vi "Main.vi"(8 "error in":errorcluster, 11 "DS TCP Server in":refnum<class "DS TCP Server.lvclass">) -> (0 "error out":errorcluster, 3 "DS TCP Server out":refnum<class "DS TCP Server.lvclass">)   [LabVIEW 2017, in "DS TCP Server.lvlib" / "DS TCP Server.lvclass"]
doc: "The <b>Queued Message Handler</b> of the Worker that owns this VI."
uses:
  DS TCP Server.lvclass
  C:/Program Files (x86)/National Instruments/LabVIEW 2017/vi.lib/addons/_Workers/Library/Classes/Worker/Worker.lvclass
  DS TCP Server.lvclass/DS TCP Server.ctl
  Initialization Data.ctl
  Response Cases.ctl
  <vilib>/addons/_Workers/Library/Case Label.ctl
  rqp_Send Data to Debug Client.ctl
  Common VIs/DC_UID.ctl
  <vilib>/addons/_Workers/Library/Classes/Message/Priority.ctl
  rqp_Start Listening.ctl
  <vilib>/addons/_Workers/Library/Classes/Message Queue/Message Queue.lvclass
  DS TCP Listener/rqp_Listen for Connections.ctl
  rqp_Message Log Ready.ctl
  Common VIs/Message Log ID.ctl
  Message Log Data.ctl
  rqp_Message Log Exited.ctl
  rsp_Server Port Open.ctl
  rsp_Connection Notify.ctl
  <vilib>/Utility/error.llb/Error Cluster From Error Code.vi
  <vilib>/ErrorRing/Error Ring.xnode
  DS TCP Listener/DS TCP Listener.lvclass
  <vilib>/addons/_Workers/Library/Workers.lvlib
  DS TCP Read/DS TCP Read.lvclass
  <vilib>/addons/_Workers/Library/Classes/Message/Message.lvclass
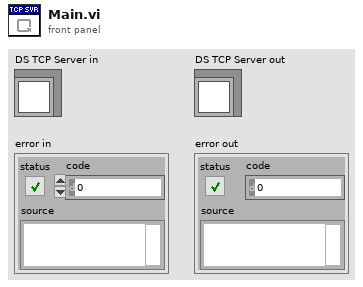
[diagram p1: front panel]
types:
  T1 = typedef "DS TCP Server.lvlib/DS TCP Server.lvclass/Initialization Data.ctl" = cluster{"Response Cases":T2}
  T2 = typedef "DS TCP Server.lvlib/DS TCP Server.lvclass/Response Cases.ctl" = cluster{"Server Port Open":T3, "Connection Notify":T3, "Incompatible DC Connection":T3}
  T3 = typedef "Workers.lvlib/Case Label.ctl" = string
  T4 = typedef "DS TCP Server.lvlib/DS TCP Server.lvclass/rqp_Send Data to Debug Client.ctl" = cluster{"DC_UID":T5, "String to send":string}
  T5 = typedef "DC_UID.ctl" = string
  T6 = typedef "Workers.lvlib/Message.lvclass/Priority.ctl" = enum16{"Low", "Normal", "High"}
  T7 = typedef "DS TCP Server.lvlib/DS TCP Listener.lvclass/rqp_Listen for Connections.ctl" = cluster{"Server Name":string, "Port":u16}
  T8 = typedef "DS TCP Server.lvlib/DS TCP Server.lvclass/rqp_Start Listening.ctl" = cluster{"Server Name":string, "Port":u16, "App Manager Q":refnum<class "Message Queue.lvclass">}
  T9 = typedef "DS TCP Server.lvlib/DS TCP Server.lvclass/rqp_Message Log Ready.ctl" = cluster{"Message Log Q":refnum<class "Message Queue.lvclass">, "Message Log ID":T10, "DC_UID":T5}
  T10 = typedef "Message Log ID.ctl" = cluster{"Head Worker ID":string, "IP Address":string}
  T11 = typedef "DS TCP Server.lvlib/DS TCP Server.lvclass/Message Log Data.ctl" = cluster{"Message Log Q":refnum<class "Message Queue.lvclass">, "Message Log ID":T10, "DC_UID":T5}
  T12 = typedef "DS TCP Server.lvlib/DS TCP Server.lvclass/rqp_Message Log Exited.ctl" = cluster{"DC_UID":T5}
  T13 = typedef "DS TCP Server.lvlib/DS TCP Server.lvclass/rsp_Server Port Open.ctl" = cluster{"Port":u16}
  T14 = typedef "DS TCP Server.lvlib/DS TCP Server.lvclass/rsp_Connection Notify.ctl" = cluster{"Connected?":bool, "DC_UID":T5, "Message Priority":T6, "IP Address":string}
  T15 = typedef "DS TCP Server.lvlib/DS TCP Server.lvclass/Connection ID.ctl" = cluster{"Connection Ref":refnum<k5>, "DC_UID":T5, "Message Priority":T6, "IP Address":string}
  T16 = typedef "DS TCP Server.lvlib/DS TCP Listener.lvclass/rsp_Add Listener.ctl" = cluster{"listener ID":refnum<k5>, "Port":u16}
  T17 = typedef "DS TCP Server.lvlib/DS TCP Read.lvclass/rsp_Connection Lost.ctl" = cluster{"connection ID out":refnum<k5>, "Message Queue":refnum<class "Message Queue.lvclass">}
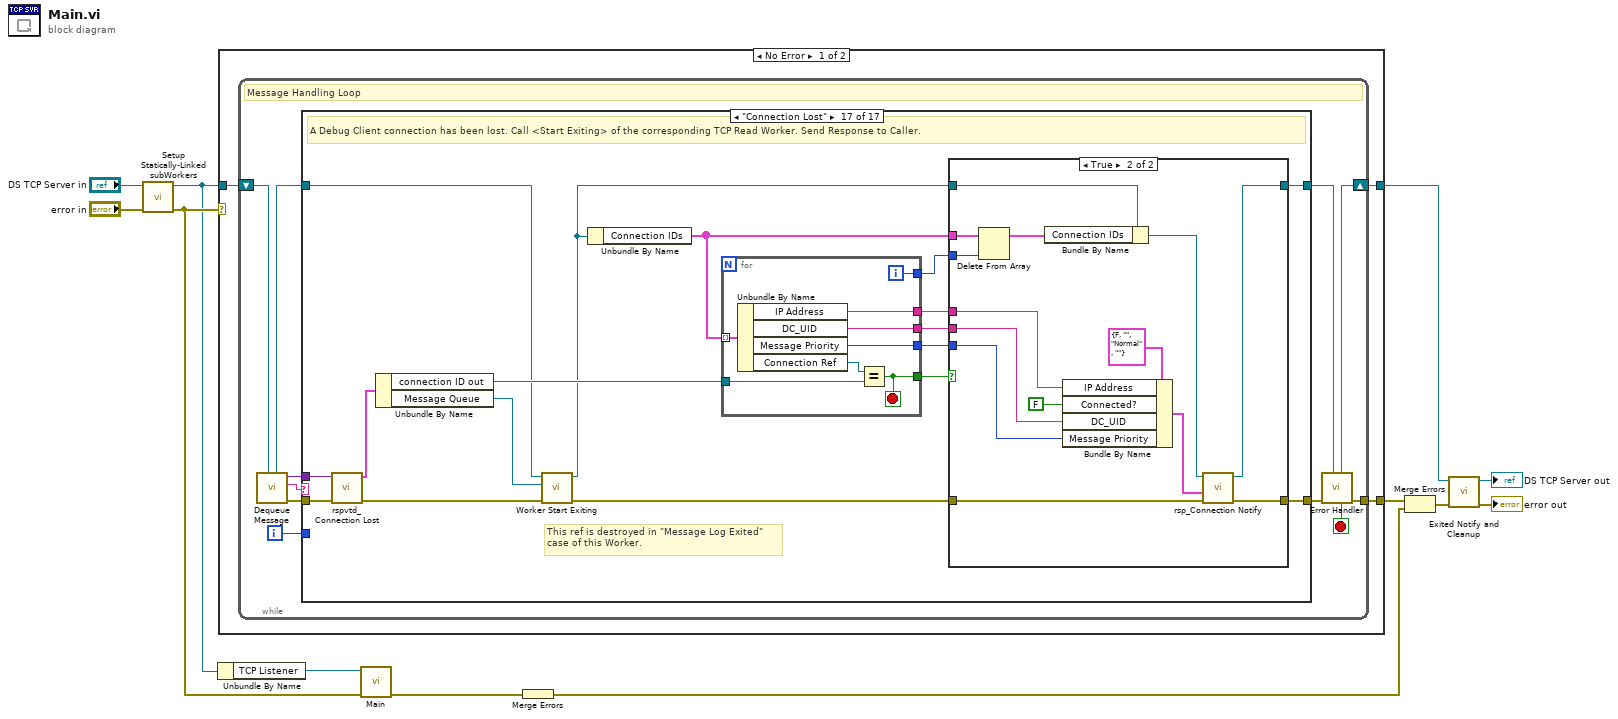
[diagram p0: block diagram]
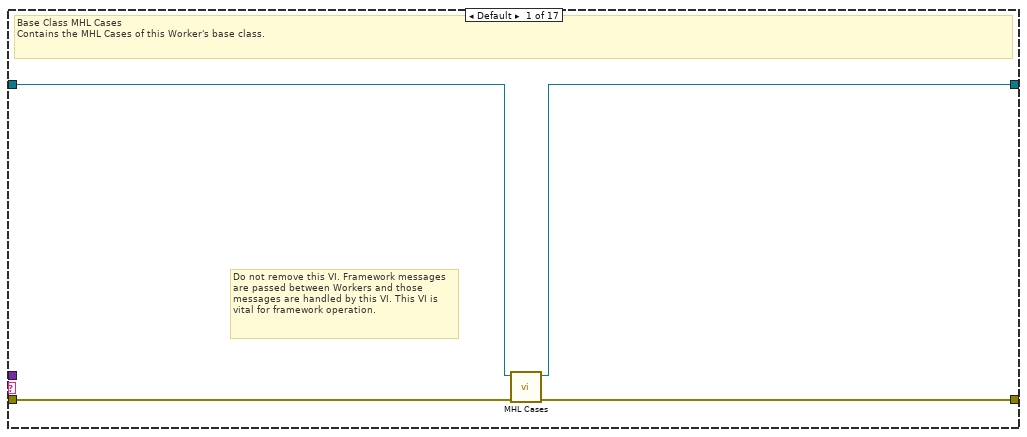
[diagram p2: hidden frame]
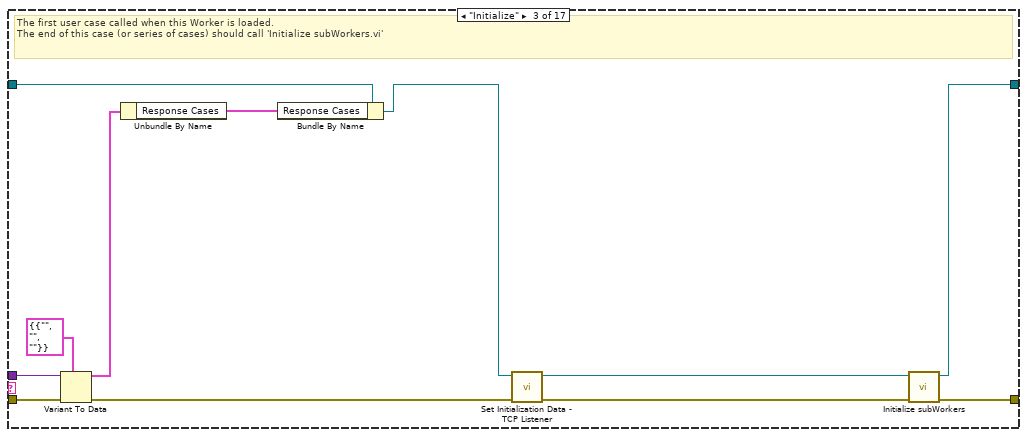
[diagram p4: hidden frame]
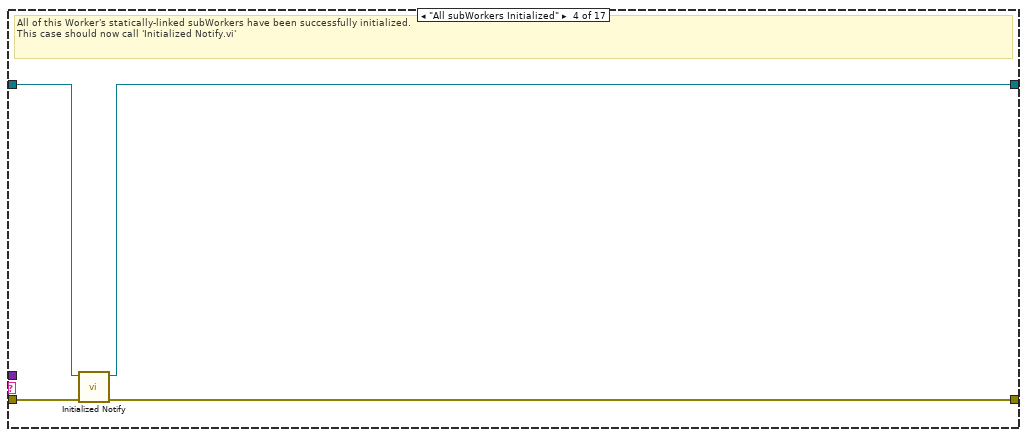
[diagram p5: hidden frame]
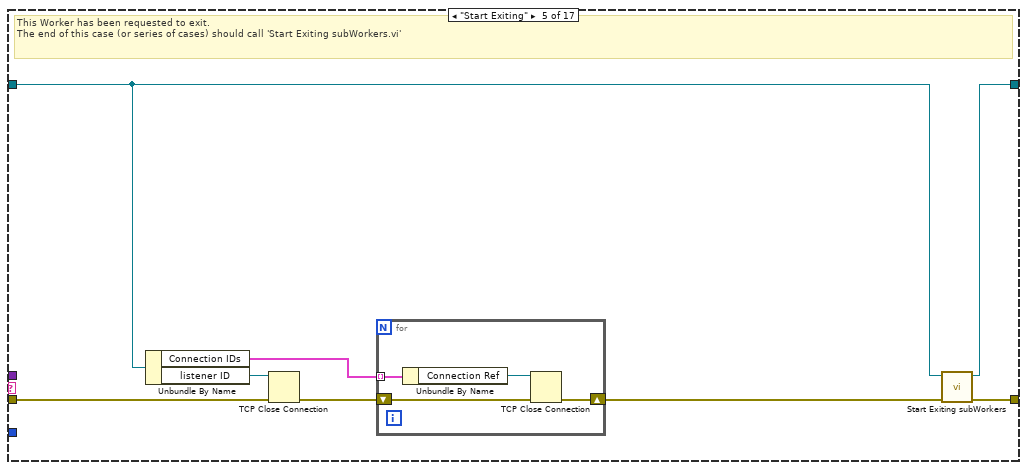
[diagram p6: hidden frame]
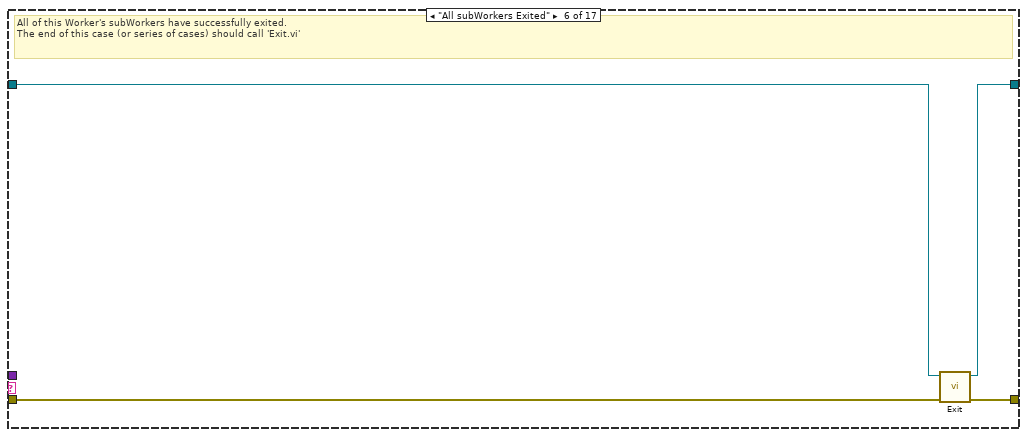
[diagram p7: hidden frame]
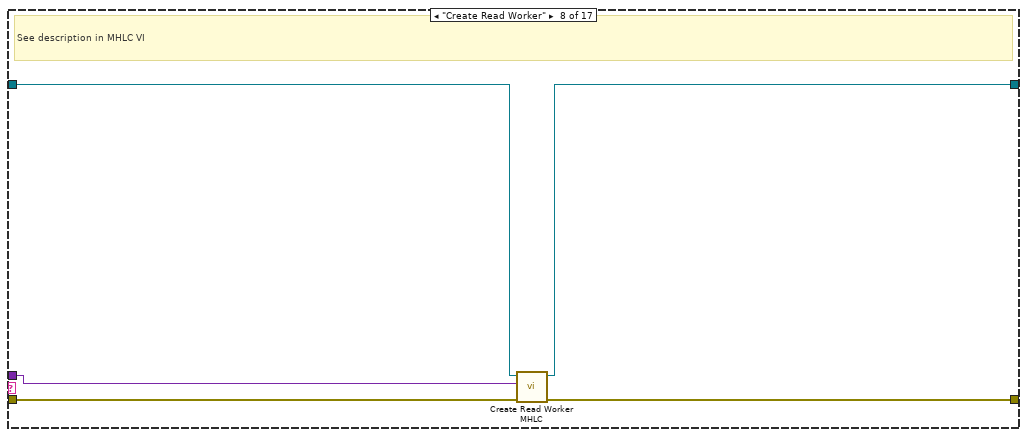
[diagram p9: hidden frame]
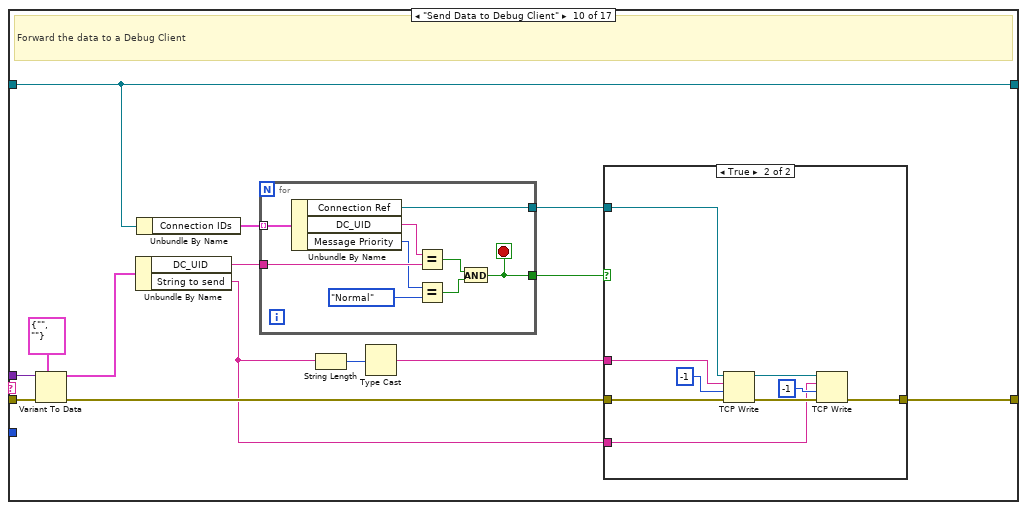
[diagram p11: hidden frame]
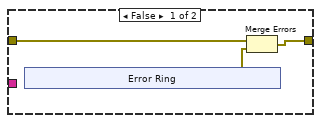
[diagram p12: hidden frame]
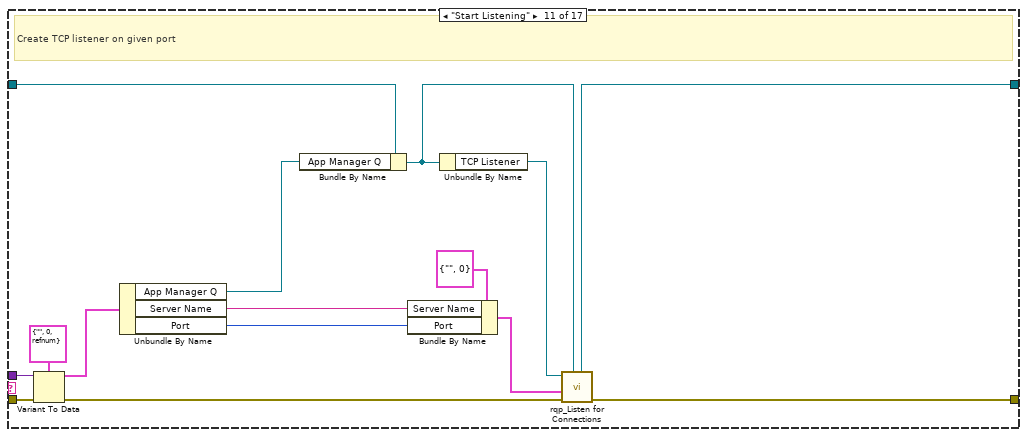
[diagram p13: hidden frame]
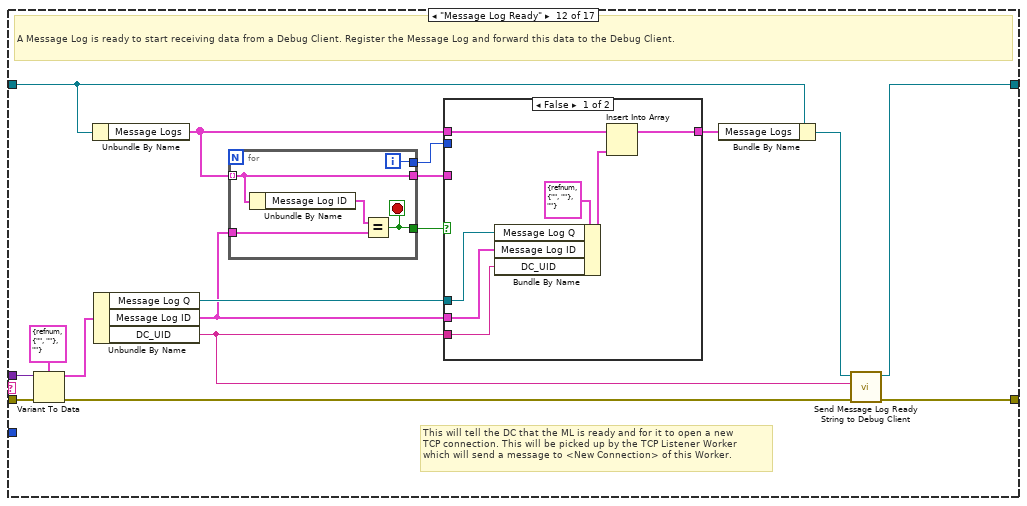
[diagram p14: hidden frame]
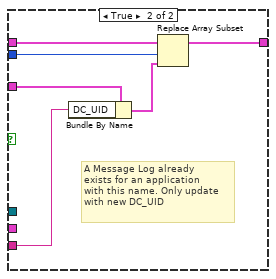
[diagram p15: hidden frame]
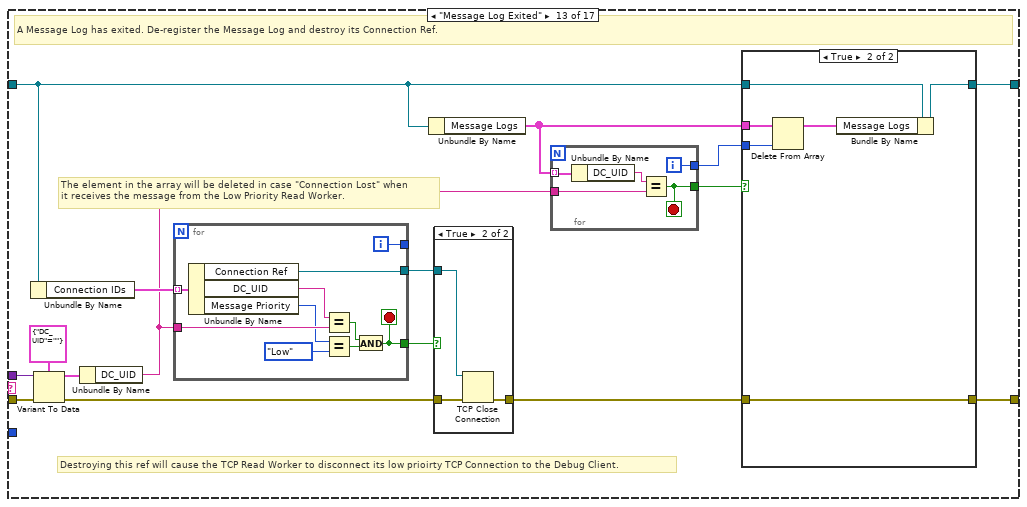
[diagram p16: hidden frame]
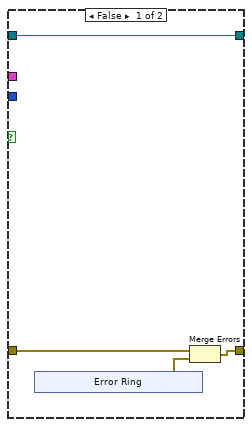
[diagram p17: hidden frame]
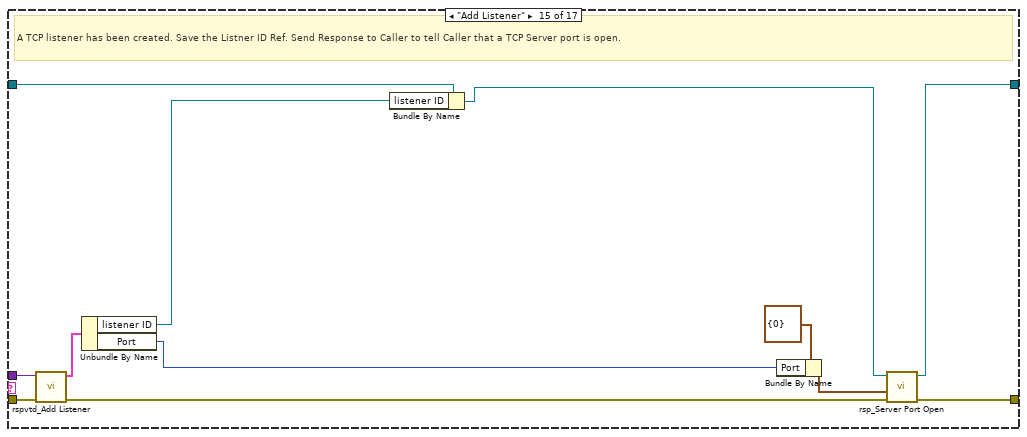
[diagram p20: hidden frame]
diagram:
  n1 = call "Setup Statically-Linked subWorkers.vi"("error in"="error in", "TCP Server in"="DS TCP Server in") -> ("error out"=w10:errorcluster, "TCP Server out"=w6:refnum<class "DS TCP Server.lvclass">)  [unwired: 8 in]
  n2 = Unbundle By Name(w6) -> ("TCP Listener"=w1:refnum<class "DS TCP Listener.lvclass">)
  n3 = case shown="No Error" w10 {
    tunnel: w6 -> [w15 w282]
    tunnel: [w13 w283] -> w9
    tunnel: [w14 w281] -> w11
    selector: w10 -> [_ w284]
    frame No Error {
      n4 = while {
        shift-right: [w24] -> w14
        shift-left: w15 -> [w26]
        tunnel: [w25] -> w13
        i -> [w17]
        stop <- w18 stop-if-true
        # "Message Handling Loop"
        n5 = call-dynamic "Dequeue Message.vi"("Worker"=w26) -> ("error out"=w23:errorcluster, "Case out"=w19:string, "Data out"=w16:variant, "Worker out"=w21:refnum<class "DS TCP Server.lvclass">)  [unwired: 6 in, 1 out]
        n6 = case "Worker MHL Case Structure (DO NOT CHANGE LABEL NAME)" shown="\"Connection Lost\"" w19 {
          tunnel: w23 -> [w30 w31 w42 w48 w54 w64 w66 w71 w73 w84 w128 w145 w179 w215 w225 w229 w239]
          tunnel: [w29 w31 w44 w46 w56 w63 w66 w69 w73 w77 w123 w140 w167 w215 w223 w230 w245] -> w22
          tunnel: w21 -> [w28 w32 w35 w47 w53 w61 w65 w67 w72 w82 w121 w138 w169 w214 w227 w232 w235]
          tunnel: [w27 w32 w43 w45 w55 w62 w65 w68 w72 w82 w122 w139 w170 w214 w224 w231 w244] -> w20
          tunnel: w17 -> [_ _ _ _ _ _ _ _ _ _ _ _ _ _ _ _ _]
          tunnel: w16 -> [_ _ w37 _ _ _ _ w70 _ w83 w125 w142 w177 _ w226 w228 w246]
          frame Default {
            # "Do not remove this VI. Framework messages are passed between Workers and those messages are handled by this VI. This VI is vital for framework operation."
            # "Base Class MHL Cases\nContains the MHL Cases of this Worker's base class."
            n7 = call-dynamic "MHL Cases.vi"("error in"=w30, "Worker in"=w28) -> ("error out"=w29:errorcluster, "Worker out"=w27:refnum<class "DS TCP Server.lvclass">)  [unwired: 8 in]
          }
          frame "------------ FRAMEWORK CASES -----------" {
            # "Start of Workers Framework Cases"
          }
          frame "Initialize" {
            # "The first user case called when this Worker is loaded.\nThe end of this case (or series of cases) should call 'Initialize subWorkers.vi'"
            n8 = Variant To Data(error in=w42, type=T1 {"Response Cases"={"Server Port Open"="", "Connection Notify"="", "Incompatible DC Connection"=""}} ("Initialization Data"), Variant=w37) -> (data=w34:T1, error out=w39:errorcluster)
            n9 = Unbundle By Name(w34) -> ("Response Cases"=w36:T2)
            n10 = Bundle By Name(cluster=w35, "Response Cases"=w36) -> (w33:refnum<class "DS TCP Server.lvclass">)
            n11 = call "Set Initialization Data - TCP Listener.vi"("error in"=w39, "TCP Server in"=w33) -> ("error out"=w41:errorcluster, "TCP Server out"=w40:refnum<class "DS TCP Server.lvclass">)  [unwired: 8 in]
            n12 = call-dynamic "Initialize subWorkers.vi"("error in"=w41, "Worker"=w40) -> ("error out"=w44:errorcluster, "dup Worker out"=w43:refnum<class "DS TCP Server.lvclass">)  [unwired: 8 in]
          }
          frame "All subWorkers Initialized" {
            # "All of this Worker's statically-linked subWorkers have been successfully initialized.\nThis case should now call 'Initialized Notify.vi'"
            n13 = call-dynamic "Initialized Notify.vi"("error in"=w48, "Worker"=w47) -> ("error out"=w46:errorcluster, "dup Worker out"=w45:refnum<class "DS TCP Server.lvclass">)  [unwired: 8 in]
          }
          frame "Start Exiting" {
            # "This Worker has been requested to exit. \nThe end of this case (or series of cases) should call 'Start Exiting subWorkers.vi'"
            n14 = Unbundle By Name(w53) -> ("Connection IDs"=w51:T15[], "listener ID"=w52:refnum<k5>)
            n15 = TCP Close Connection(connection ID=w52, error in (no error)=w54) -> (error out=w50:errorcluster)  [unwired: 1 in, 1 out]
            n16 = for {
              shift-right: [w59] -> w49
              shift-left: w50 -> [w60]
              tunnel: w51 -> [w58] mode=indexing
              n17 = Unbundle By Name(w58) -> ("Connection Ref"=w57:refnum<k5>)
              n18 = TCP Close Connection(connection ID=w57, error in (no error)=w60) -> (error out=w59:errorcluster)  [unwired: 1 in, 1 out]
            }
            n19 = call-dynamic "Start Exiting subWorkers.vi"("error_in"=w49, "Worker"=w53) -> ("error out"=w56:errorcluster, "dup Worker out"=w55:refnum<class "DS TCP Server.lvclass">)  [unwired: 8 in]
          }
          frame "All subWorkers Exited" {
            # "All of this Worker's subWorkers have successfully exited. \nThe end of this case (or series of cases) should call 'Exit.vi'"
            n20 = call-dynamic "Exit.vi"("error_in"=w64, "Worker"=w61) -> ("error out"=w63:errorcluster, "dup Worker out"=w62:refnum<class "DS TCP Server.lvclass">)  [unwired: 8 in]
          }
          frame "------------- LOCAL API CASES -------------" {
            # "Start of Workers Local API Cases"
          }
          frame "Create Read Worker" {
            # "See description in MHLC VI"
            n21 = call "Create Read Worker MHLC.vi"("error in (no error)"=w71, "Data in"=w70, "TCPServer in"=w67) -> ("error out"=w69:errorcluster, "TCPServer out"=w68:refnum<class "DS TCP Server.lvclass">)  [unwired: 7 in]
          }
          frame "------------- PUBLIC API CASES -------------" {
            # "Start of Public API Cases"
          }
          frame "Send Data to Debug Client" {
            # "Forward the data to a Debug Client"
            n22 = Variant To Data(error in=w84, type=T4 {"DC_UID"="", "String to send"=""} ("Data"), Variant=w83) -> (data=w81:T4, error out=w78:errorcluster)
            n23 = Unbundle By Name(w81) -> ("DC_UID"=w80:T5, "String to send"=w75:string)
            n24 = Unbundle By Name(w82) -> ("Connection IDs"=w87:T15[])
            n25 = for {
              tunnel: w87 -> [w113] mode=indexing
              tunnel: w80 -> [w111]
              tunnel: [w110] -> w74
              tunnel: [w105] -> w79
              stop <- w105 stop-if-true
              n26 = Unbundle By Name(w113) -> ("Connection Ref"=w110:refnum<k5>, "DC_UID"=w112:T5, "Message Priority"=w109:T6)
              n27 = Equal?(x=w112, y=w111) -> (x = y?=w107:bool)
              n28 = Equal?(x=w109, y=Priority."Normal") -> (x = y?=w106:bool)
              n29 = And(x=w107, y=w106) -> (x .and. y?=w105:bool)
            }
            n30 = String Length(string=w75) -> (length=w86:i32)
            n31 = Type Cast(x=w86) -> (*(type *) &x=w76:string)  [unwired: 1 in]
            n32 = case shown="True" w79 {
              tunnel: w78 -> [w90 w100]
              tunnel: [w89 w99] -> w77
              tunnel: w76 -> [_ w98]
              tunnel: w75 -> [_ w97]
              tunnel: w74 -> [_ w96]
              frame False {
                n33 = xnode "Error Ring"() -> ("error out"=w88:errorcluster)
                n34 = Merge Errors(w90, w88) -> (w89:errorcluster)
              }
              frame True {
                n35 = TCP Write(connection ID=w96, data in=w98, error in (no error)=w100, 9:-1 ("timeout ms (25000)")) -> (connection ID out=w102:refnum<k5>, error out=w101:errorcluster)  [unwired: 1 out]
                n36 = TCP Write(connection ID=w102, data in=w97, error in (no error)=w101, 9:-1 ("timeout ms (25000)")) -> (error out=w99:errorcluster)  [unwired: 2 out]
              }
            }
          }
          frame "Start Listening" {
            # "Create TCP listener on given port"
            n37 = Variant To Data(error in=w128, type=T8 {"Server Name"="", "Port"=0, "App Manager Q"=refnum} ("Data"), Variant=w125) -> (data=w124:T8, error out=w127:errorcluster)
            n38 = Unbundle By Name(w124) -> ("App Manager Q"=w114:refnum<class "Message Queue.lvclass">, "Server Name"=w117:string, "Port"=w116:u16)
            n39 = Bundle By Name(cluster=w121, "App Manager Q"=w114) -> (w115:refnum<class "DS TCP Server.lvclass">)
            n40 = Bundle By Name(cluster=T7 {"Server Name"="", "Port"=0} ("Data"), "Server Name"=w117, "Port"=w116) -> (w118:T7)
            n41 = Unbundle By Name(w115) -> ("TCP Listener"=w120:refnum<class "DS TCP Listener.lvclass">)
            n42 = call "rqp_Listen for Connections.vi"("Caller in"=w115, "error in"=w127, "Data"=w118, "DS TCP Listener in"=w120) -> ("error out"=w123:errorcluster, "dup Caller out"=w122:refnum<class "DS TCP Server.lvclass">)  [unwired: 5 in, 1 out]
          }
          frame "Message Log Ready" {
            # "This will tell the DC that the ML is ready and for it to open a new\nTCP connection. This will be picked up by the TCP Listener Worker\nwhich will send a message to <New Connection> of this Worker."
            # "A Message Log is ready to start receiving data from a Debug Client. Register the Message Log and forward this data to the Debug Client."
            n43 = Variant To Data(error in=w145, type=T9 {"Message Log Q"=refnum, "Message Log ID"={"Head Worker ID"="", "IP Address"=""}, "DC_UID"=""} ("Data"), Variant=w142) -> (data=w141:T9, error out=w144:errorcluster)
            n44 = Unbundle By Name(w138) -> ("Message Logs"=w134:T11[])
            n45 = Unbundle By Name(w141) -> ("Message Log Q"=w137:refnum<class "Message Queue.lvclass">, "Message Log ID"=w133:T10, "DC_UID"=w131:T5)
            n46 = for {
              tunnel: w134 -> [w159] mode=indexing
              tunnel: w133 -> [w162]
              tunnel: [w161] -> w132
              tunnel: [w160] -> w129
              tunnel: [w159] -> w130
              i -> [w160]
              stop <- w161 stop-if-true
              n47 = Unbundle By Name(w159) -> ("Message Log ID"=w163:T10)
              n48 = Equal?(x=w163, y=w162) -> (x = y?=w161:bool)
            }
            n49 = case shown="False" w132 {
              tunnel: w137 -> [w150 _]
              tunnel: [w149 w157] -> w135
              tunnel: w134 -> [w148 w158]
              tunnel: w133 -> [w147 _]
              tunnel: w131 -> [w146 w155]
              tunnel: w130 -> [_ w156]
              tunnel: w129 -> [_ w153]
              frame False {
                n50 = Bundle By Name(cluster=T11 {"Message Log Q"=refnum, "Message Log ID"={"Head Worker ID"="", "IP Address"=""}, "DC_UID"=""} ("new element/subarray"), "Message Log Q"=w150, "Message Log ID"=w147, "DC_UID"=w146) -> (w151:T11)
                n51 = Insert Into Array(array=w148, new element=w151) -> (w149:T11[])  [unwired: 1 in]
              }
              frame True {
                # "A Message Log already\nexists for an application\nwith this name. Only update\nwith new DC_UID"
                n52 = Bundle By Name(cluster=w156, "DC_UID"=w155) -> (w154:T11)
                n53 = Replace Array Subset(array=w158, new element=w154, index=w153) -> (w157:T11[])
              }
            }
            n54 = Bundle By Name(cluster=w138, "Message Logs"=w135) -> (w136:refnum<class "DS TCP Server.lvclass">)
            n55 = call "Send Message Log Ready String to Debug Client.vi"("error in (no error)"=w144, "DC_UID"=w131, "DS TCP Server in"=w136) -> ("error out"=w140:errorcluster, "DS TCP Server out"=w139:refnum<class "DS TCP Server.lvclass">)  [unwired: 7 in]
          }
          frame "Message Log Exited" {
            # "Destroying this ref will cause the TCP Read Worker to disconnect its low prioirty TCP Connection to the Debug Client."
            # "The element in the array will be deleted in case \"Connection Lost\" when\nit receives the message from the Low Priority Read Worker."
            # "A Message Log has exited. De-register the Message Log and destroy its Connection Ref."
            n56 = Unbundle By Name(w169) -> ("Connection IDs"=w173:T15[])
            n57 = Variant To Data(error in=w179, type=T12 {"DC_UID"=""} ("Data"), Variant=w177) -> (data=w176:T12, error out=w174:errorcluster)
            n58 = Unbundle By Name(w176) -> ("DC_UID"=w171:T5)
            n59 = for {
              tunnel: w173 -> [w213] mode=indexing
              tunnel: [w204] -> w175
              tunnel: [w211] -> w172
              tunnel: w171 -> [w210]
              tunnel: [w209] -> _
              i -> [w209]
              stop <- w204 stop-if-true
              n60 = Unbundle By Name(w213) -> ("Connection Ref"=w211:refnum<k5>, "DC_UID"=w212:T5, "Message Priority"=w208:T6)
              n61 = Equal?(x=w212, y=w210) -> (x = y?=w205:bool)
              n62 = Equal?(x=w208, y=Priority."Low") -> (x = y?=w206:bool)
              n63 = And(x=w205, y=w206) -> (x .and. y?=w204:bool)
            }
            n64 = Unbundle By Name(w169) -> ("Message Logs"=w165:T11[])
            n65 = case shown="True" w175 {
              tunnel: w174 -> [w200 w203]
              tunnel: [w200 w201] -> w166
              tunnel: w172 -> [_ w202]
              frame False {
              }
              frame True {
                n66 = TCP Close Connection(connection ID=w202, error in (no error)=w203) -> (error out=w201:errorcluster)  [unwired: 1 in, 1 out]
              }
            }
            n67 = for {
              tunnel: w165 -> [w199] mode=indexing
              tunnel: w171 -> [w197]
              tunnel: [w196] -> w168
              tunnel: [w195] -> w164
              i -> [w195]
              stop <- w196 stop-if-true
              n68 = Unbundle By Name(w199) -> ("DC_UID"=w198:T5)
              n69 = Equal?(x=w198, y=w197) -> (x = y?=w196:bool)
            }
            n70 = case shown="True" w168 {
              tunnel: [w183 w190] -> w170
              tunnel: w169 -> [w183 w194]
              tunnel: [w181 w193] -> w167
              tunnel: w166 -> [w182 w193]
              tunnel: w165 -> [_ w192]
              tunnel: w164 -> [_ w191]
              frame False {
                n71 = xnode "Error Ring"() -> ("error out"=w180:errorcluster)
                n72 = Merge Errors(w182, w180) -> (w181:errorcluster)
              }
              frame True {
                n73 = Delete From Array(array=w192, index=w191) -> (array with subset deleted=w189:T11[])  [unwired: 1 in, 1 out]
                n74 = Bundle By Name(cluster=w194, "Message Logs"=w189) -> (w190:refnum<class "DS TCP Server.lvclass">)
              }
            }
          }
          frame "------------- RESPONSE CASES -------------" {
          }
          frame "Add Listener" {
            # "A TCP listener has been created. Save the Listner ID Ref. Send Response to Caller to tell Caller that a TCP Server port is open."
            n75 = call "rspvtd_Add Listener.vi"("error in"=w225, "Data in"=w226) -> ("error out"=w222:errorcluster, "Data out"=w220:T16)  [unwired: 8 in]
            n76 = Unbundle By Name(w220) -> ("listener ID"=w219:refnum<k5>, "Port"=w216:u16)
            n77 = Bundle By Name(cluster=w227, "listener ID"=w219) -> (w221:refnum<class "DS TCP Server.lvclass">)
            n78 = Bundle By Name(cluster=T13 {"Port"=0} ("Cluster"), "Port"=w216) -> (w217:T13)
            n79 = call "rsp_Server Port Open.vi"("error in"=w222, "Placeholder"=w217, "DS TCP Server in"=w221) -> ("error out"=w223:errorcluster, "dup DS TCP Server out"=w224:refnum<class "DS TCP Server.lvclass">)  [unwired: 7 in]
          }
          frame "New Connection" {
            # "See description in MHLC VI"
            n80 = call "New Connection MHLC.vi"("error in (no error)"=w229, "Data in"=w228, "TCPServer in"=w232) -> ("error out"=w230:errorcluster, "TCPServer out"=w231:refnum<class "DS TCP Server.lvclass">)  [unwired: 7 in]
          }
          frame "Connection Lost" {
            # "This ref is destroyed in \"Message Log Exited\"\ncase of this Worker."
            # "A Debug Client connection has been lost. Call <Start Exiting> of the corresponding TCP Read Worker. Send Response to Caller."
            n81 = call "rspvtd_Connection Lost.vi"("error in"=w239, "Data in"=w246) -> ("error out"=w249:errorcluster, "Data out"=w238:T17)  [unwired: 8 in]
            n82 = Unbundle By Name(w238) -> ("connection ID out"=w237:refnum<k5>, "Message Queue"=w233:refnum<class "Message Queue.lvclass">)
            n83 = call-dynamic "Worker Start Exiting.vi"("error_in"=w249, "Message Queue"=w233, "Worker"=w235) -> ("error out"=w236:errorcluster, "dup Worker out"=w234:refnum<class "DS TCP Server.lvclass">)  [unwired: 7 in]
            n84 = Unbundle By Name(w234) -> ("Connection IDs"=w248:T15[])
            n85 = for {
              tunnel: w248 -> [w280] mode=indexing
              tunnel: w237 -> [w278]
              tunnel: [w277] -> w247
              tunnel: [w276] -> w242
              tunnel: [w275] -> w243
              tunnel: [w274] -> w241
              tunnel: [w273] -> w240
              i -> [w277]
              stop <- w274 stop-if-true
              n86 = Unbundle By Name(w280) -> ("IP Address"=w273:string, "DC_UID"=w275:T5, "Message Priority"=w276:T6, "Connection Ref"=w279:refnum<k5>)
              n87 = Equal?(x=w279, y=w278) -> (x = y?=w274:bool)
            }
            n88 = case shown="True" w241 {
              tunnel: w236 -> [w252 w272]
              tunnel: w234 -> [w253 w271]
              tunnel: w248 -> [_ w268]
              tunnel: w247 -> [_ w267]
              tunnel: [w251 w266] -> w245
              tunnel: [w253 w265] -> w244
              tunnel: w243 -> [_ w261]
              tunnel: w242 -> [_ w260]
              tunnel: w240 -> [_ w259]
              frame False {
                n89 = xnode "Error Ring"() -> ("error out"=w250:errorcluster)
                n90 = Merge Errors(w252, w250) -> (w251:errorcluster)
              }
              frame True {
                n91 = Delete From Array(array=w268, index=w267) -> (array with subset deleted=w269:T15[])  [unwired: 1 in, 1 out]
                n92 = Bundle By Name(cluster=w271, "Connection IDs"=w269) -> (w270:refnum<class "DS TCP Server.lvclass">)
                n93 = Bundle By Name(cluster=T14 {"Connected?"=FALSE, "DC_UID"="", "Message Priority"=enum."Normal", "IP Address"=""} ("Data in"), "IP Address"=w259, "Connected?"=FALSE, "DC_UID"=w261, "Message Priority"=w260) -> (w262:T14)
                n94 = call "rsp_Connection Notify.vi"("error in"=w272, "Data in"=w262, "DS TCP Server in"=w270) -> ("error out"=w266:errorcluster, "dup DS TCP Server out"=w265:refnum<class "DS TCP Server.lvclass">)  [unwired: 7 in]
              }
            }
          }
        }
        n95 = call-dynamic "Error Handler.vi"("Worker"=w20, "error_in"=w22) -> ("error out"=w25:errorcluster, "Stop Loop"=w18:bool, "Worker out"=w24:refnum<class "DS TCP Server.lvclass">)  [unwired: 7 in]
      }
    }
    frame Error {
      n96 = call-dynamic "Error Handler.vi"("Worker"=w282, "error_in"=w284) -> ("error out"=w283:errorcluster, "Worker out"=w281:refnum<class "DS TCP Server.lvclass">)  [unwired: 7 in, 1 out]
    }
  }
  n97 = call-dynamic "Main.vi"("error in"=w10, "TCP Listener in"=w1) -> ("error out"=w3:errorcluster)  [unwired: 8 in, 1 out]
  n98 = Merge Errors(w3) -> (w2:errorcluster)
  n99 = Merge Errors(w9, w2) -> (w12:errorcluster)
  n100 = call-dynamic "Exited Notify and Cleanup.vi"("error_in"=w12, "Worker"=w11) -> ("error out"=→"error out":errorcluster, "dup Worker out"=→"DS TCP Server out":refnum<class "DS TCP Server.lvclass">)  [unwired: 8 in]
